vi "Open.vi"(8 "error in (no error)":errorcluster, 9 "Collect? (T)":bool=TRUE, 10 "VI Path":path, 11 "Thread Name":string) -> (0 "error out":errorcluster, 2 "Generic VI Reference":refnum<vi>, 3 "VI Reference":variant)   [LabVIEW 2021, in "Thread.lvlib"]
uses:
  Thread.lvlib
  Cache Action.ctl
  <vilib>/Utility/error.llb/Error Cluster From Error Code.vi
  <vilib>/ErrorRing/Error Ring.xnode
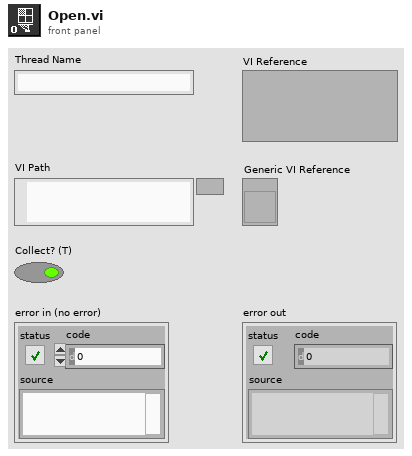
[diagram p1: front panel]
types:
  T1 = typedef "Thread.lvlib/Cache Action.ctl" = enum8{"noop", "get", "add", "remove", "remove_by_ref"}
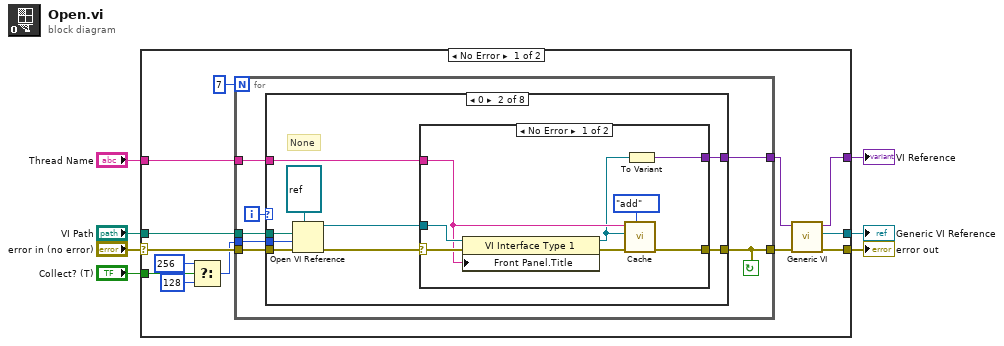
[diagram p0: block diagram]
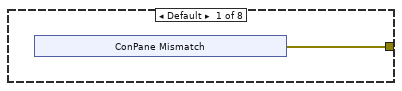
[diagram p2: hidden frame]
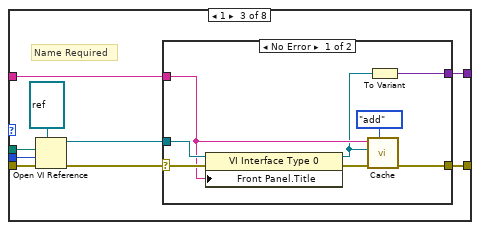
[diagram p4: hidden frame]
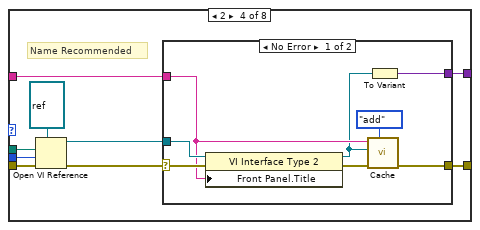
[diagram p6: hidden frame]
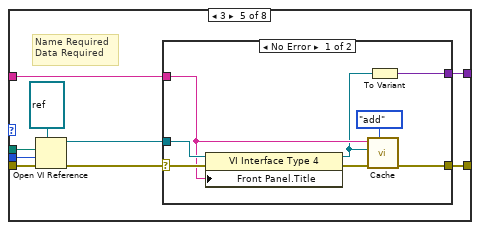
[diagram p8: hidden frame]
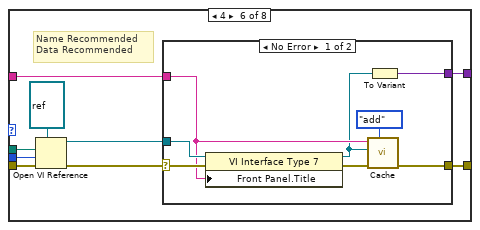
[diagram p10: hidden frame]
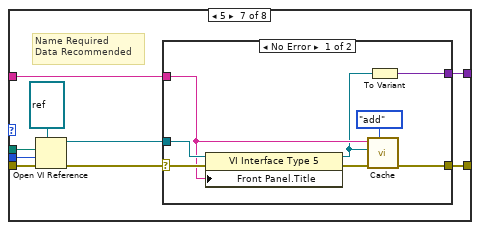
[diagram p12: hidden frame]
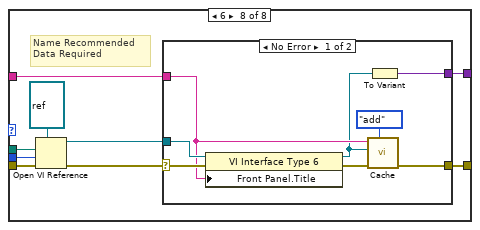
[diagram p14: hidden frame]
diagram:
  n1 = case shown="No Error" "error in (no error)" {
    selector: "error in (no error)" -> [w19 w159]
    tunnel: "VI Path" -> [w18 _]
    tunnel: "Collect? (T)" -> [w16 _]
    tunnel: "Thread Name" -> [w14 _]
    tunnel: [w11 w159] -> w3
    tunnel: [w9 _] -> w2
    tunnel: [w8 _] -> w1
    frame No Error {
      n2 = Select(t=256 ("options"), s=w16, f=128 ("options")) -> (s? t:f=w17:i32)
      n3 = for {
        N: 7 -> [_]
        tunnel: w18 -> [w26]
        tunnel: w17 -> [w25]
        tunnel: w14 -> [w24]
        tunnel: [w23] -> w10
        tunnel: w19 -> [w27]
        tunnel: [w21] -> w12
        i -> [w22]
        stop <- w21 continue-if-true
        n4 = case shown="0" w22 {
          tunnel: w27 -> [_ w41 w59 w77 w95 w113 w131 w149]
          tunnel: w26 -> [_ w39 w57 w75 w93 w111 w129 w147]
          tunnel: w25 -> [_ w38 w56 w74 w92 w110 w128 w146]
          tunnel: w24 -> [_ w36 w54 w72 w90 w108 w126 w144]
          tunnel: [w28 w35 w53 w71 w89 w107 w125 w143] -> w21
          tunnel: [_ w34 w52 w70 w88 w106 w124 w142] -> w23
          frame Default {
            n5 = xnode "ConPane Mismatch"() -> ("error out"=w28:errorcluster)
          }
          frame 0 {
            # "None"
            n6 = Open VI Reference(type specifier VI Refnum (for type only)=refnum<vi> refnum ("VI Refnum"), vi path=w39, options=w38, error in (no error)=w41) -> (vi reference=w37:refnum<vi>, error out=w40:errorcluster)  [unwired: 2 in]
            n7 = case shown="No Error" w40 {
              selector: w40 -> [w49 w50]
              tunnel: w37 -> [w48 _]
              tunnel: w36 -> [w46 _]
              tunnel: [w45 w50] -> w35
              tunnel: [w43 _] -> w34
              frame No Error {
                n8 = property class="VI Interface Type 1"(reference=w48, error in=w49, "Front Panel.Title"=w46) -> (reference out=w44:refnum<vi>, error out=w47:errorcluster)
                n9 = call "Cache.vi"("Action"=Cache_Action."add", "error in (no error)"=w47, "VI in"=w44, "Thread Name"=w46) -> ("error out"=w45:errorcluster)  [unwired: 3 in, 4 out]
                n10 = To Variant(anything=w44) -> (Variant=w43:variant)
              }
              frame Error {
              }
            }
          }
          frame 1 {
            # "Name Required"
            n11 = Open VI Reference(type specifier VI Refnum (for type only)=refnum<vi> refnum ("VI Refnum"), vi path=w57, options=w56, error in (no error)=w59) -> (vi reference=w55:refnum<vi>, error out=w58:errorcluster)  [unwired: 2 in]
            n12 = case shown="No Error" w58 {
              selector: w58 -> [w67 w68]
              tunnel: w55 -> [w66 _]
              tunnel: w54 -> [w64 _]
              tunnel: [w63 w68] -> w53
              tunnel: [w61 _] -> w52
              frame No Error {
                n13 = property class="VI Interface Type 0"(reference=w66, error in=w67, "Front Panel.Title"=w64) -> (reference out=w62:refnum<vi>, error out=w65:errorcluster)
                n14 = call "Cache.vi"("Action"=Cache_Action."add", "error in (no error)"=w65, "VI in"=w62, "Thread Name"=w64) -> ("error out"=w63:errorcluster)  [unwired: 3 in, 4 out]
                n15 = To Variant(anything=w62) -> (Variant=w61:variant)
              }
              frame Error {
              }
            }
          }
          frame 2 {
            # "Name Recommended"
            n16 = Open VI Reference(type specifier VI Refnum (for type only)=refnum<vi> refnum ("VI Refnum"), vi path=w75, options=w74, error in (no error)=w77) -> (vi reference=w73:refnum<vi>, error out=w76:errorcluster)  [unwired: 2 in]
            n17 = case shown="No Error" w76 {
              selector: w76 -> [w85 w86]
              tunnel: w73 -> [w84 _]
              tunnel: w72 -> [w82 _]
              tunnel: [w81 w86] -> w71
              tunnel: [w79 _] -> w70
              frame No Error {
                n18 = property class="VI Interface Type 2"(reference=w84, error in=w85, "Front Panel.Title"=w82) -> (reference out=w80:refnum<vi>, error out=w83:errorcluster)
                n19 = call "Cache.vi"("Action"=Cache_Action."add", "error in (no error)"=w83, "VI in"=w80, "Thread Name"=w82) -> ("error out"=w81:errorcluster)  [unwired: 3 in, 4 out]
                n20 = To Variant(anything=w80) -> (Variant=w79:variant)
              }
              frame Error {
              }
            }
          }
          frame 3 {
            # "Name Required\nData Required"
            n21 = Open VI Reference(type specifier VI Refnum (for type only)=refnum<vi> refnum ("VI Refnum"), vi path=w93, options=w92, error in (no error)=w95) -> (vi reference=w91:refnum<vi>, error out=w94:errorcluster)  [unwired: 2 in]
            n22 = case shown="No Error" w94 {
              selector: w94 -> [w103 w104]
              tunnel: w91 -> [w102 _]
              tunnel: w90 -> [w100 _]
              tunnel: [w99 w104] -> w89
              tunnel: [w97 _] -> w88
              frame No Error {
                n23 = property class="VI Interface Type 4"(reference=w102, error in=w103, "Front Panel.Title"=w100) -> (reference out=w98:refnum<vi>, error out=w101:errorcluster)
                n24 = call "Cache.vi"("Action"=Cache_Action."add", "error in (no error)"=w101, "VI in"=w98, "Thread Name"=w100) -> ("error out"=w99:errorcluster)  [unwired: 3 in, 4 out]
                n25 = To Variant(anything=w98) -> (Variant=w97:variant)
              }
              frame Error {
              }
            }
          }
          frame 4 {
            # "Name Recommended\nData Recommended"
            n26 = Open VI Reference(type specifier VI Refnum (for type only)=refnum<vi> refnum ("VI Refnum"), vi path=w111, options=w110, error in (no error)=w113) -> (vi reference=w109:refnum<vi>, error out=w112:errorcluster)  [unwired: 2 in]
            n27 = case shown="No Error" w112 {
              selector: w112 -> [w121 w122]
              tunnel: w109 -> [w120 _]
              tunnel: w108 -> [w118 _]
              tunnel: [w117 w122] -> w107
              tunnel: [w115 _] -> w106
              frame No Error {
                n28 = property class="VI Interface Type 7"(reference=w120, error in=w121, "Front Panel.Title"=w118) -> (reference out=w116:refnum<vi>, error out=w119:errorcluster)
                n29 = call "Cache.vi"("Action"=Cache_Action."add", "error in (no error)"=w119, "VI in"=w116, "Thread Name"=w118) -> ("error out"=w117:errorcluster)  [unwired: 3 in, 4 out]
                n30 = To Variant(anything=w116) -> (Variant=w115:variant)
              }
              frame Error {
              }
            }
          }
          frame 5 {
            # "Name Required\nData Recommended"
            n31 = Open VI Reference(type specifier VI Refnum (for type only)=refnum<vi> refnum ("VI Refnum"), vi path=w129, options=w128, error in (no error)=w131) -> (vi reference=w127:refnum<vi>, error out=w130:errorcluster)  [unwired: 2 in]
            n32 = case shown="No Error" w130 {
              selector: w130 -> [w139 w140]
              tunnel: w127 -> [w138 _]
              tunnel: w126 -> [w136 _]
              tunnel: [w135 w140] -> w125
              tunnel: [w133 _] -> w124
              frame No Error {
                n33 = property class="VI Interface Type 5"(reference=w138, error in=w139, "Front Panel.Title"=w136) -> (reference out=w134:refnum<vi>, error out=w137:errorcluster)
                n34 = call "Cache.vi"("Action"=Cache_Action."add", "error in (no error)"=w137, "VI in"=w134, "Thread Name"=w136) -> ("error out"=w135:errorcluster)  [unwired: 3 in, 4 out]
                n35 = To Variant(anything=w134) -> (Variant=w133:variant)
              }
              frame Error {
              }
            }
          }
          frame 6 {
            # "Name Recommended\nData Required"
            n36 = Open VI Reference(type specifier VI Refnum (for type only)=refnum<vi> refnum ("VI Refnum"), vi path=w147, options=w146, error in (no error)=w149) -> (vi reference=w145:refnum<vi>, error out=w148:errorcluster)  [unwired: 2 in]
            n37 = case shown="No Error" w148 {
              selector: w148 -> [w157 w158]
              tunnel: w145 -> [w156 _]
              tunnel: w144 -> [w154 _]
              tunnel: [w153 w158] -> w143
              tunnel: [w151 _] -> w142
              frame No Error {
                n38 = property class="VI Interface Type 6"(reference=w156, error in=w157, "Front Panel.Title"=w154) -> (reference out=w152:refnum<vi>, error out=w155:errorcluster)
                n39 = call "Cache.vi"("Action"=Cache_Action."add", "error in (no error)"=w155, "VI in"=w152, "Thread Name"=w154) -> ("error out"=w153:errorcluster)  [unwired: 3 in, 4 out]
                n40 = To Variant(anything=w152) -> (Variant=w151:variant)
              }
              frame Error {
              }
            }
          }
        }
      }
      n41 = call "Generic VI.vi"("error in (no error)"=w12, "VI Reference in"=w10) -> ("error out"=w11:errorcluster, "Generic VI Reference"=w8:refnum<vi>, "VI Reference out"=w9:variant)  [unwired: 7 in]
    }
    frame Error {
    }
  }
  "error out" <- w3
  "Generic VI Reference" <- w1
  "VI Reference" <- w2
